vi "RampGenerator.vi"(2 "Number of Positions":u16=100 min=1 step=1, 3 "End  (um)":dbl=10.0 min=0.0 max=100.0 step=0.2 format="%.3f", 4 "Start  (um)":dbl min=0.0 max=100.0 step=0.5 format="%.3f") -> (0 "Array":dbl[](array[numeric]) format="%.2f")   [LabVIEW 2015]
panel:
  # "Generates a linear ramp from Start to End (inclusive).\nThis example is used as a SubVI in the provided scanning examples."
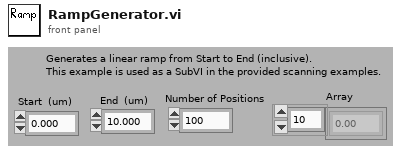
[diagram p1: front panel]
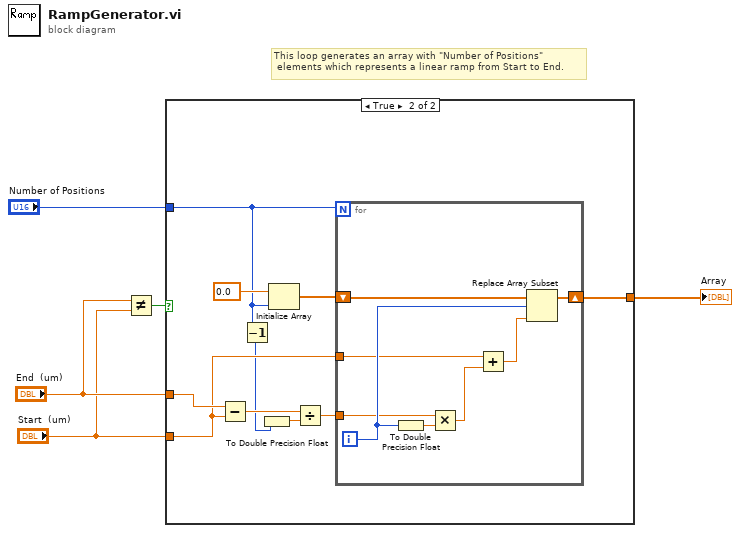
[diagram p0: block diagram]
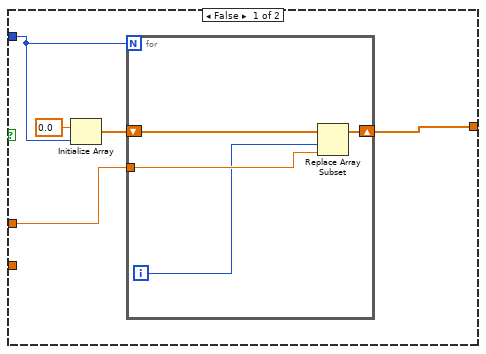
[diagram p2: hidden frame]
diagram:
  # "This loop generates an array with \"Number of Positions\"\n elements which represents a linear ramp from Start to End."
  n1 = Not Equal?(x="End  (um)", y="Start  (um)") -> (x != y?=w4:bool)
  n2 = case shown="True" w4 {
    tunnel: "End  (um)" -> [w8 w22]
    tunnel: [w7 w18] -> w5
    tunnel: "Start  (um)" -> [_ w17]
    tunnel: "Number of Positions" -> [w6 w15]
    frame False {
      n3 = Initialize Array(0.0, w6) -> (w9:dbl[])
      n4 = for {
        N: w6 -> [_]
        shift-right: [w13] -> w7
        shift-left: w9 -> [w14]
        tunnel: w8 -> [w12]
        i -> [w11]
        n5 = Replace Array Subset(array=w14, new element=w12, index=w11) -> (w13:dbl[])
      }
    }
    frame True {
      n6 = Subtract(x=w22, y=w17) -> (x-y=w21:dbl)
      n7 = Decrement(x=w15) -> (x-1=w16:u16)
      n8 = To Double Precision Float(number=w16) -> (double precision float=w20:dbl)
      n9 = Initialize Array(0.0, w15) -> (w23:dbl[])
      n10 = Divide(x=w21, y=w20) -> (x/y=w19:dbl)
      n11 = for {
        N: w15 -> [_]
        shift-right: [w31] -> w18
        shift-left: w23 -> [w32]
        tunnel: w19 -> [w28]
        tunnel: w17 -> [w25]
        i -> [w29]
        n12 = To Double Precision Float(number=w29) -> (double precision float=w30:dbl)
        n13 = Multiply(x=w28, y=w30) -> (x*y=w27:dbl)
        n14 = Add(x=w25, y=w27) -> (x+y=w26:dbl)
        n15 = Replace Array Subset(array=w32, new element=w26, index=w29) -> (w31:dbl[])
      }
    }
  }
  "Array" <- w5
